vi "Set Enable State.vi"(8 "error in (no error)":errorcluster, 10 "Enable":bool, 11 "Abs_Value.lvclass in":refnum<class "Abs_Value.lvclass">) -> (0 "error out":errorcluster, 3 "Abs_Value.lvclass out":refnum<class "Abs_Value.lvclass">)   [LabVIEW 2021, in "Fault-Injection_Type.lvclass"]
uses:
  Support/Interfaces/Type/Fault-Injection_Type.lvclass
  <vilib>/TSA/Abstract Data Classes/Abs_Types/Value/Abs_Value.lvclass
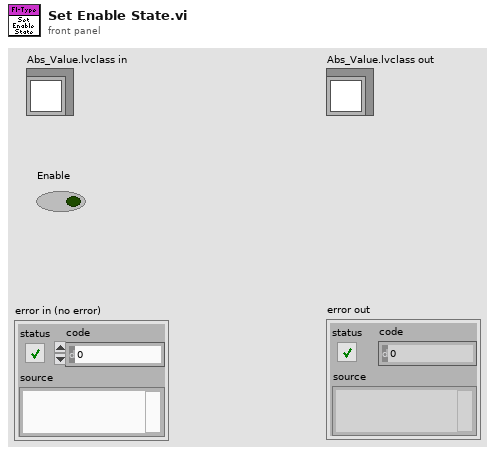
[diagram p1: front panel]
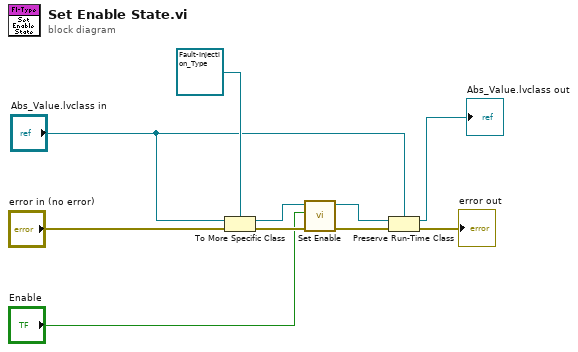
[diagram p0: block diagram]
diagram:
  n1 = To More Specific Class(target class=refnum<class "Fault-Injection_Type.lvclass"> refnum ("Fault-Injection_Type.lvclass"), reference="Abs_Value.lvclass in", error in="error in (no error)") -> (specific class reference=w9:refnum<class "Fault-Injection_Type.lvclass">, error out=w10:errorcluster)
  n2 = call-dynamic "Set Enable.vi"("error in (no error)"=w10, "Enable"="Enable", "Fault-Insertion_Type in"=w9) -> ("error out"=w7:errorcluster, "Fault-Insertion_Type out"=w3:refnum<class "Fault-Injection_Type.lvclass">)  [unwired: 7 in]
  n3 = Preserve Run-Time Class(object in=w3, error in=w7, 2:"Abs_Value.lvclass in") -> (object out=→"Abs_Value.lvclass out":refnum<class "Abs_Value.lvclass">, error out=→"error out":errorcluster)
